vi "Open Logic VI.vi"(11 "error in (no error)":errorcluster) -> (15 "error out":errorcluster)   [LabVIEW 2021, in "Converter.lvlib"]
uses:
  Converter.lvlib
  Path Functions/Path Functions.lvlib
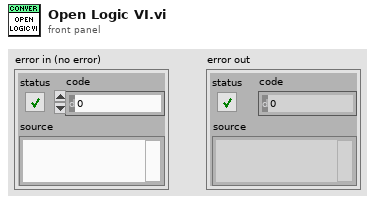
[diagram p1: front panel]
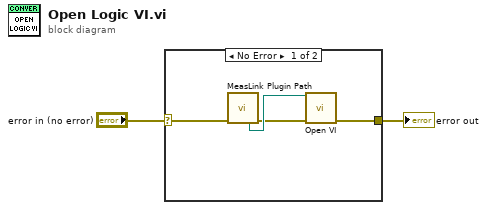
[diagram p0: block diagram]
diagram:
  n1 = case shown="No Error" "error in (no error)" {
    selector: "error in (no error)" -> [w6 w7]
    tunnel: [w3 w7] -> w1
    frame No Error {
      n2 = call "MeasLink Plugin Path.vi"("error in (no error)"=w6) -> ("Logic VI Path"=w5:path, "error out"=w4:errorcluster)  [unwired: 2 in, 11 out]
      n3 = call "Open VI.vi"("Logic VI Path"=w5, "error in (no error)"=w4) -> ("error out"=w3:errorcluster)  [unwired: 13 in]
    }
    frame Error {
    }
  }
  "error out" <- w1
